vi "readWithTimeout.vi"(8 "error in":errorcluster, 10 "timeOut":u32, 11 "Port":refnum<visa-resource-name>) -> (0 "error out":errorcluster, 2 "String":string, 3 "Port out":refnum<visa-resource-name>)   [LabVIEW 2018]
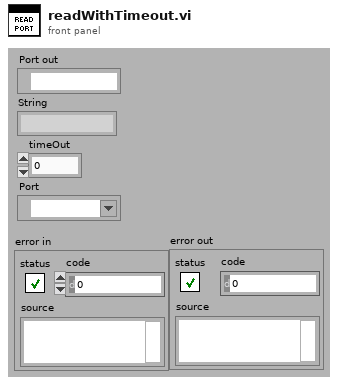
[diagram p1: front panel]
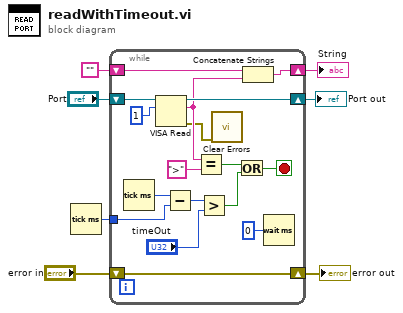
[diagram p0: block diagram]
diagram:
  n1 = Tick Count (ms)() -> (millisecond timer value=w6:u32)
  n2 = while {
    shift-left: "" -> [w23]
    shift-right: [w24] -> w3
    shift-right: [w20] -> w4
    shift-left: "Port" -> [w21]
    tunnel: w6 -> [w16]
    shift-right: [w9] -> w1
    shift-left: "error in" -> [w9]
    stop <- w12 stop-if-true
    n3 = Tick Count (ms)() -> (millisecond timer value=w17:u32)
    n4 = VISA Read(VISA resource name=w21, byte count=u32 1) -> (VISA resource name out=w20:refnum<visa-resource-name>, read buffer=w19:string, error out=w10:errorcluster)  [unwired: 1 in, 1 out]
    n5 = Subtract(x=w17, y=w16) -> (x-y=w15:u32)
    n6 = Equal?(x=w19, y=">") -> (x = y?=w13:bool)
    n7 = Greater?(x=w15, y="timeOut") -> (0:w11:bool)
    n8 = call <vilib>:"Clear Errors.vi"("error in (no error)"=w10) -> ()  [unwired: 5 in, 2 out]
    n9 = Or(x=w13, y=w11) -> (x .or. y?=w12:bool)
    n10 = Concatenate Strings(w23, w19) -> (w24:string)
    n11 = Wait (ms)(milliseconds to wait=u32 0) -> ()  [unwired: 1 out]
  }
  "Port out" <- w4
  "String" <- w3
  "error out" <- w1
